vi "Configure Gamma Magnitude-Phase Pairs.vi"(8 "error in (no error)":errorcluster, 9 "Magnitude Phase Pairs":dbl[](array[numeric]), 10 "Gamma Table Name (\"DEFAULT\")":string="DEFAULT", 11 "VISA resource name":refnum<visa-resource-name>) -> (0 "error out":errorcluster, 3 "VISA resource name out":refnum<visa-resource-name>)   [LabVIEW 2014, in "Agilent U2000 Series.lvlib"]
doc: "Sets the magnitude-phase pairs for the source gamma for the currently selected gamma table. \n\nNote:\nThis VI is only applicable for U2040 X-Series."
uses:
  Agilent U2000 Series.lvlib
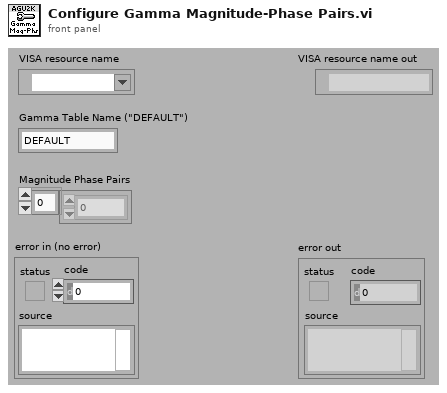
[diagram p1: front panel]
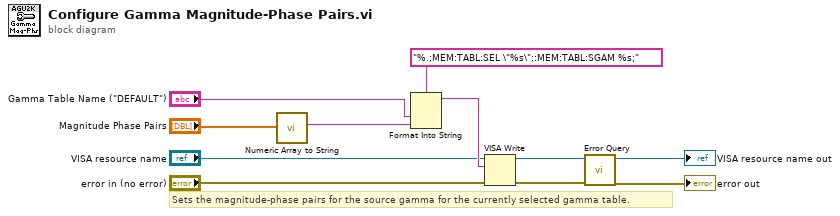
[diagram p0: block diagram]
diagram:
  # "Sets the magnitude-phase pairs for the source gamma for the currently selected gamma table."
  n1 = call "Numeric Array to String.vi"("List Data"="Magnitude Phase Pairs") -> ("Result String"=w2:string)  [unwired: 10 out]
  n2 = Format Into String(format string="%.;MEM:TABL:SEL \"%s\";:MEM:TABL:SGAM %s;", "Gamma Table Name (\"DEFAULT\")", w2) -> (resulting string=w10:string)  [unwired: 2 in, 1 out]
  n3 = VISA Write(VISA resource name="VISA resource name", write buffer=w10, error in (no error)="error in (no error)") -> (VISA resource name out=w7:refnum<visa-resource-name>, error out=w6:errorcluster)  [unwired: 1 out]
  n4 = call "Error Query.vi"("error in (no error)"=w6, "VISA resource name"=w7) -> ("error out"=→"error out":errorcluster, "VISA resource name out"=→"VISA resource name out":refnum<visa-resource-name>)  [unwired: 6 in, 2 out]
